vi "Dashboard Main.vi"() -> ()   [LabVIEW 2015]
uses:
  <vilib>/event_ctls.llb/eventvkey.ctl
  <vilib>/Rock Robotics/WPI/Dashboard/WPI_DashboardLogging Global.vi
  <vilib>/Rock Robotics/Network Tables/SD Read Number.vi
  <vilib>/Utility/config.llb/Write Key (String).vi
  <vilib>/Utility/config.llb/Write Key (I32).vi
  <vilib>/Utility/config.llb/NI_LVConfig.lvlib
panel:
  in  "TCP":refnum<k5>
  in  "Rec Mode":enum32{"Stop", "Record", "Playback"}(radio)
  in  "Vision":u16(ring) items=["Camera Off", "USB Camera SW", "USB Camera HW", "IP Camera"]
  out "Camera IP":string
  out "Image Message":string="Timeout in Camera Communications"
  in  "Dashboard Tab":T1(tab)
  out "TargetLocked":bool caption="Locked"
  out "AutoTarget":bool caption="Target\nTarget"
  out "ShooterLowPower":bool caption="Shoot Low"
  out "LSOverride":bool caption="LS OVR"
  out "PickupMotor":bool caption="Pickup"
  out "ShooterMotor":bool caption="Shooter"
  out "PTO":bool
  out "High":bool caption="High Gear"
  out "Low":bool caption="Low Gear"
  in  "CompressorEnabled":bool caption="Compressor"
  out "Compressor":bool
  in  "AutoProgramSelect":u16(ring) items=["0 - No Auto Program", "1 - Drive to Defense and Stop", "2 - Cross Rough Ground", "3 - Cross Rock Wall", "4 - Shoot from Spybot Start", "5 - Test Drive with Gyro"]
  out "Low Battery":bool
  out "FMS":bool
  out "Teleop Mode":bool
  out "Auto Mode":bool
  out "Disabled":bool
  in  "Program":string
  in  "Camera Settings":T2={"Frame Rate"=30, "Compression"=30, "Size"=1} {"Frame Rate" scale=1.0..30.0; "Size" items=["640x480", "320x240", "160x120"]}
  out "Mode":T3(ring)=enum."Auto Disabled"
  in  "DB Camera Config":bool
  out "fps":dbl format="%#.1g"
  out "Mbps":dbl format="%#.1g"
  out "Mbps 2":bool
  in  "PIDEnabled":bool caption="PID Enabled"
  in  "LCD_Line_10":string caption="DB/String 0"
  in  "LCD_Line_9":string caption="DB/String 0"
  in  "LCD_Line_8":string caption="DB/String 0"
  in  "LCD_Line_7":string caption="DB/String 0"
  in  "LCD_Line_6":string caption="DB/String 0"
  in  "LCD_Line_5":string caption="DB/String 0"
  in  "LCD_Line_4":string caption="DB/String 0"
  in  "LCD_Line_3":string caption="DB/String 0"
  in  "LCD_Line_2":string caption="DB/String 0"
  in  "LCD_Line_1":string caption="DB/String 0"
  in  "PValue":dbl caption="P"
  in  "IValue":dbl caption="I"
  in  "DValue":dbl caption="D"
  in  "LowSetting":dbl caption="Low"
  in  "HighSetting":dbl caption="High"
  in  "DB/String 9":string
  in  "DB/String 8":string
  in  "DB/String 7":string
  in  "DB/String 6":string
  in  "DB/String 5":string
  in  "DB/String 4":string
  in  "DB/String 3":string
  in  "DB/String 2":string
  in  "DB/String 1":string
  in  "DB/String 0":string
  in  "DB/Slider 0":dbl(slide) scale=0.0..5.0
  in  "DB/Slider 1":dbl(slide) scale=0.0..5.0
  in  "DB/Slider 2":dbl(slide) scale=0.0..5.0
  in  "DB/Slider 3":dbl(slide) scale=0.0..5.0
  out "DB/LED 3":bool
  out "DB/LED 2":bool
  out "DB/LED 1":bool
  out "DB/LED 0":bool
  in  "DB/Button 3":bool
  in  "DB/Button 2":bool
  in  "DB/Button 1":bool
  in  "DB/Button 0":bool caption="New Name"
  in  "Test Slider":dbl(slide) scale=0.0..100.0 scale format="%#_3g"
  in  "On/Off":bool caption="Solenoid"
  in  "Test Name":u16(ring) items=["Select the test to run...", "Example Test", "-------------------------------", "List of tests is built in robot code.", "Replace with your own automated tests."]
  in  "Test Tree":string(tree)
  in  "Motor":cluster{"Value":dbl, "Enable":bool} {"Value" scale=-1.0..1.0 scale format="%#_3g"}
  out "Progress":T4 {"Test Progress" scale=0.0..100.0}
  in  "Rev/Fwd":cluster{"Forward":bool, "Reverse":bool}
  in  "Test Ring":u16(ring) items=["Monochrome", "Color"]
  in  "Listbox":i32(listbox)
  out "Tree":string(tree)
  out "Camera Image":T5(plugin-control)
  out "Boolean":bool
  # "Program:"
  # "Dashboard: 2016-06"
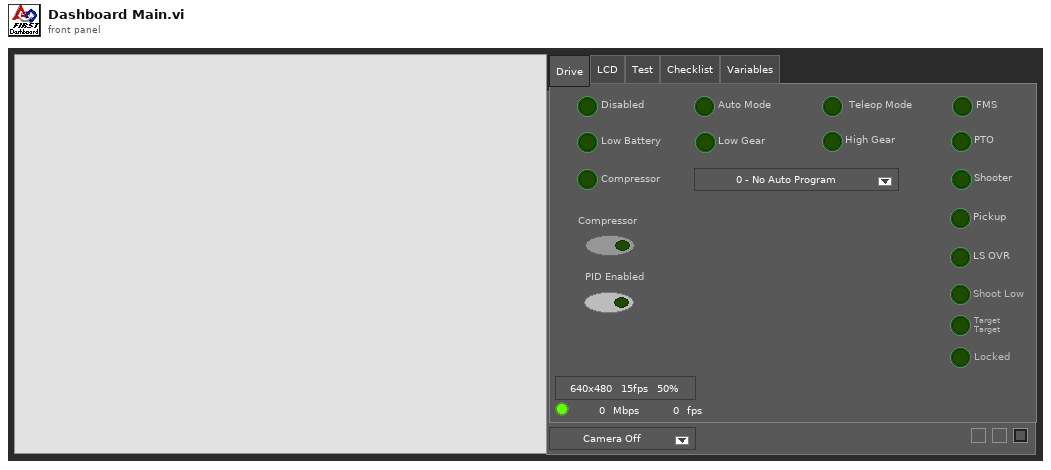
[diagram p1: front panel]
types:
  T1 = enum32{"Drive", "LCD", "Basic", "Test", "Checklist", "Variables"}
  T2 = cluster{"Frame Rate":i32, "Compression":i32, "Size":u16}
  T3 = enum8{"Tele-Op Disabled", "Tele-Op Enabled", "Auto Disabled", "Auto Enabled", "Test Disabled", "Test Enabled", "Disconnected", "No Code", "E-Stop"}
  T4 = cluster{"Test Progress":u8, "Test Progress Text":string}
  T5 = typedef "IMAQ Image.ctl" = refnum<image>
  T6 = enum32{"Drive", "Basic", "Custom", "Test", "Checklist", "Variables"}
  T7 = typedef "Image Type" = u32
  T8 = cluster{"Camera Image":refnum<vi>, "Dashboard Tab":refnum<vi>, "Boolean":refnum<vi>, "Vision":refnum<vi>, "Rec Mode":refnum<vi>, "Test Slider":refnum<vi>, "On/Off ":refnum<vi>, "Test Ring":refnum<vi>, "Rev/Fwd":refnum<vi>, "Test Name":refnum<vi>, "Motor":refnum<vi>, "Progress":refnum<vi>, "CheckList":refnum<vi>, "Tree":refnum<vi>, "Test Tree":refnum<vi>}
  T9 = cluster{"Error Strings":string, "Disable Counts":cluster{u16, u16}, "Rail Faults":cluster{u16, u16, u16}, "Robot IP":string, "DB Mode":u8, "Event Info":cluster{"Name":string, "Type":u8, "Number":u16, "Replay":u8}, "Camera Addr":string}
  T10 = cluster{"Storage":cluster{"Disk Free":u64, "RAM Block":u32, "RAM free":u32}, "CPU Utilization":cluster{"CPU % ISR":sgl, "CPU % Time Crit":sgl, "CPU % Timed Str":sgl, "CPU % High":sgl, "CPU % Above":sgl, "CPU % Normal":sgl, "CPU % Low":sgl}, "CAN":cluster{"% Bus Utilization":sgl, "Bus Off Cnt":u32, "TX_FIFO Full Cnt":u32, "Receive Error Cnt":u8, "Transmit Error Cnt":u8}, "HID":cluster{"HID Outputs":u32, "Rumble Low":u16, "Rumble High":u16}[]}
  T11 = cluster{"Status bits":cluster{"Test Mode":bool, "Autonomous":bool, "Enabled":bool, "Code Start":bool, "Brownout":bool, "Reserved 2":bool, "Reserved 3":bool, "E-Stop":bool}, "Code Trace":cluster{"Disabled":bool, "TeleOp":bool, "Auto":bool, "Test":bool}, "Controller Type":enum16{"unknown", "cRIO", "roboRio"}, "Code?":enum16{"unknown", "noCode", "code"}, "Battery V":dbl}
  T12 = cluster{"Control Bits":cluster{"TestMode":bool, "Autonomous":bool, "Enabled":bool, "FMS Present":bool, bool, bool, bool, "E-Stop":bool}, "Team Station ":u8, "Countdown":sgl, "Joystick Values":cluster{"Axes":dbl[], "Buttons":bool[], "POVs":i16[]}[]}
  T13 = cluster{"Axes":dbl[], "Buttons":bool[], "POVs":i16[]}[]
  T14 = cluster{"Axes":dbl[], "Buttons":bool[], "POVs":i16[]}
  T15 = typedef "NI_LVConfig.lvlib/Config Data RefNum.ctl" = refnum<k1>
  T16 = cluster{"Operation":enum16{"Update", "Clear"}, "Color Box":u32}[]
  T17 = typedef "eventvkey.ctl" = enum16{"ASCII", "Enter", "Return", "Shift", "Ctrl", "Alt", "Cmd", "Opt", "Caps", "NumLock", "Clear", "Break", "Up", "Down", "Left", "Right", "Insert", "Delete", "Home", "End", "PageUp", "PageDown", "Escape", "Help", "Pause", "ScrollLock", "F1", "F2", "F3", "F4", "F5", "F6", "F7", "F8", "F9", "F10", "F11", "F12", "F13", "F14", "F15", "F16", "F17", "F18", "F19", "F20", "F21", "F22", "F23", "F24", "Play", "VolumeUp", "VolumeDown", "Mute", "Two Byte Char"}
  T18 = cluster{"Image Size":bool, "Image Type":bool, "Pixel Value":bool, "ROI Information":bool, "Zoom Factor":bool}
  T19 = enum8{"Enabled", "Disabled", "Disabled and Grayed Out"}
  T20 = cluster{"Operation":enum16{"Update", "Clear"}, "Color Box":u32}
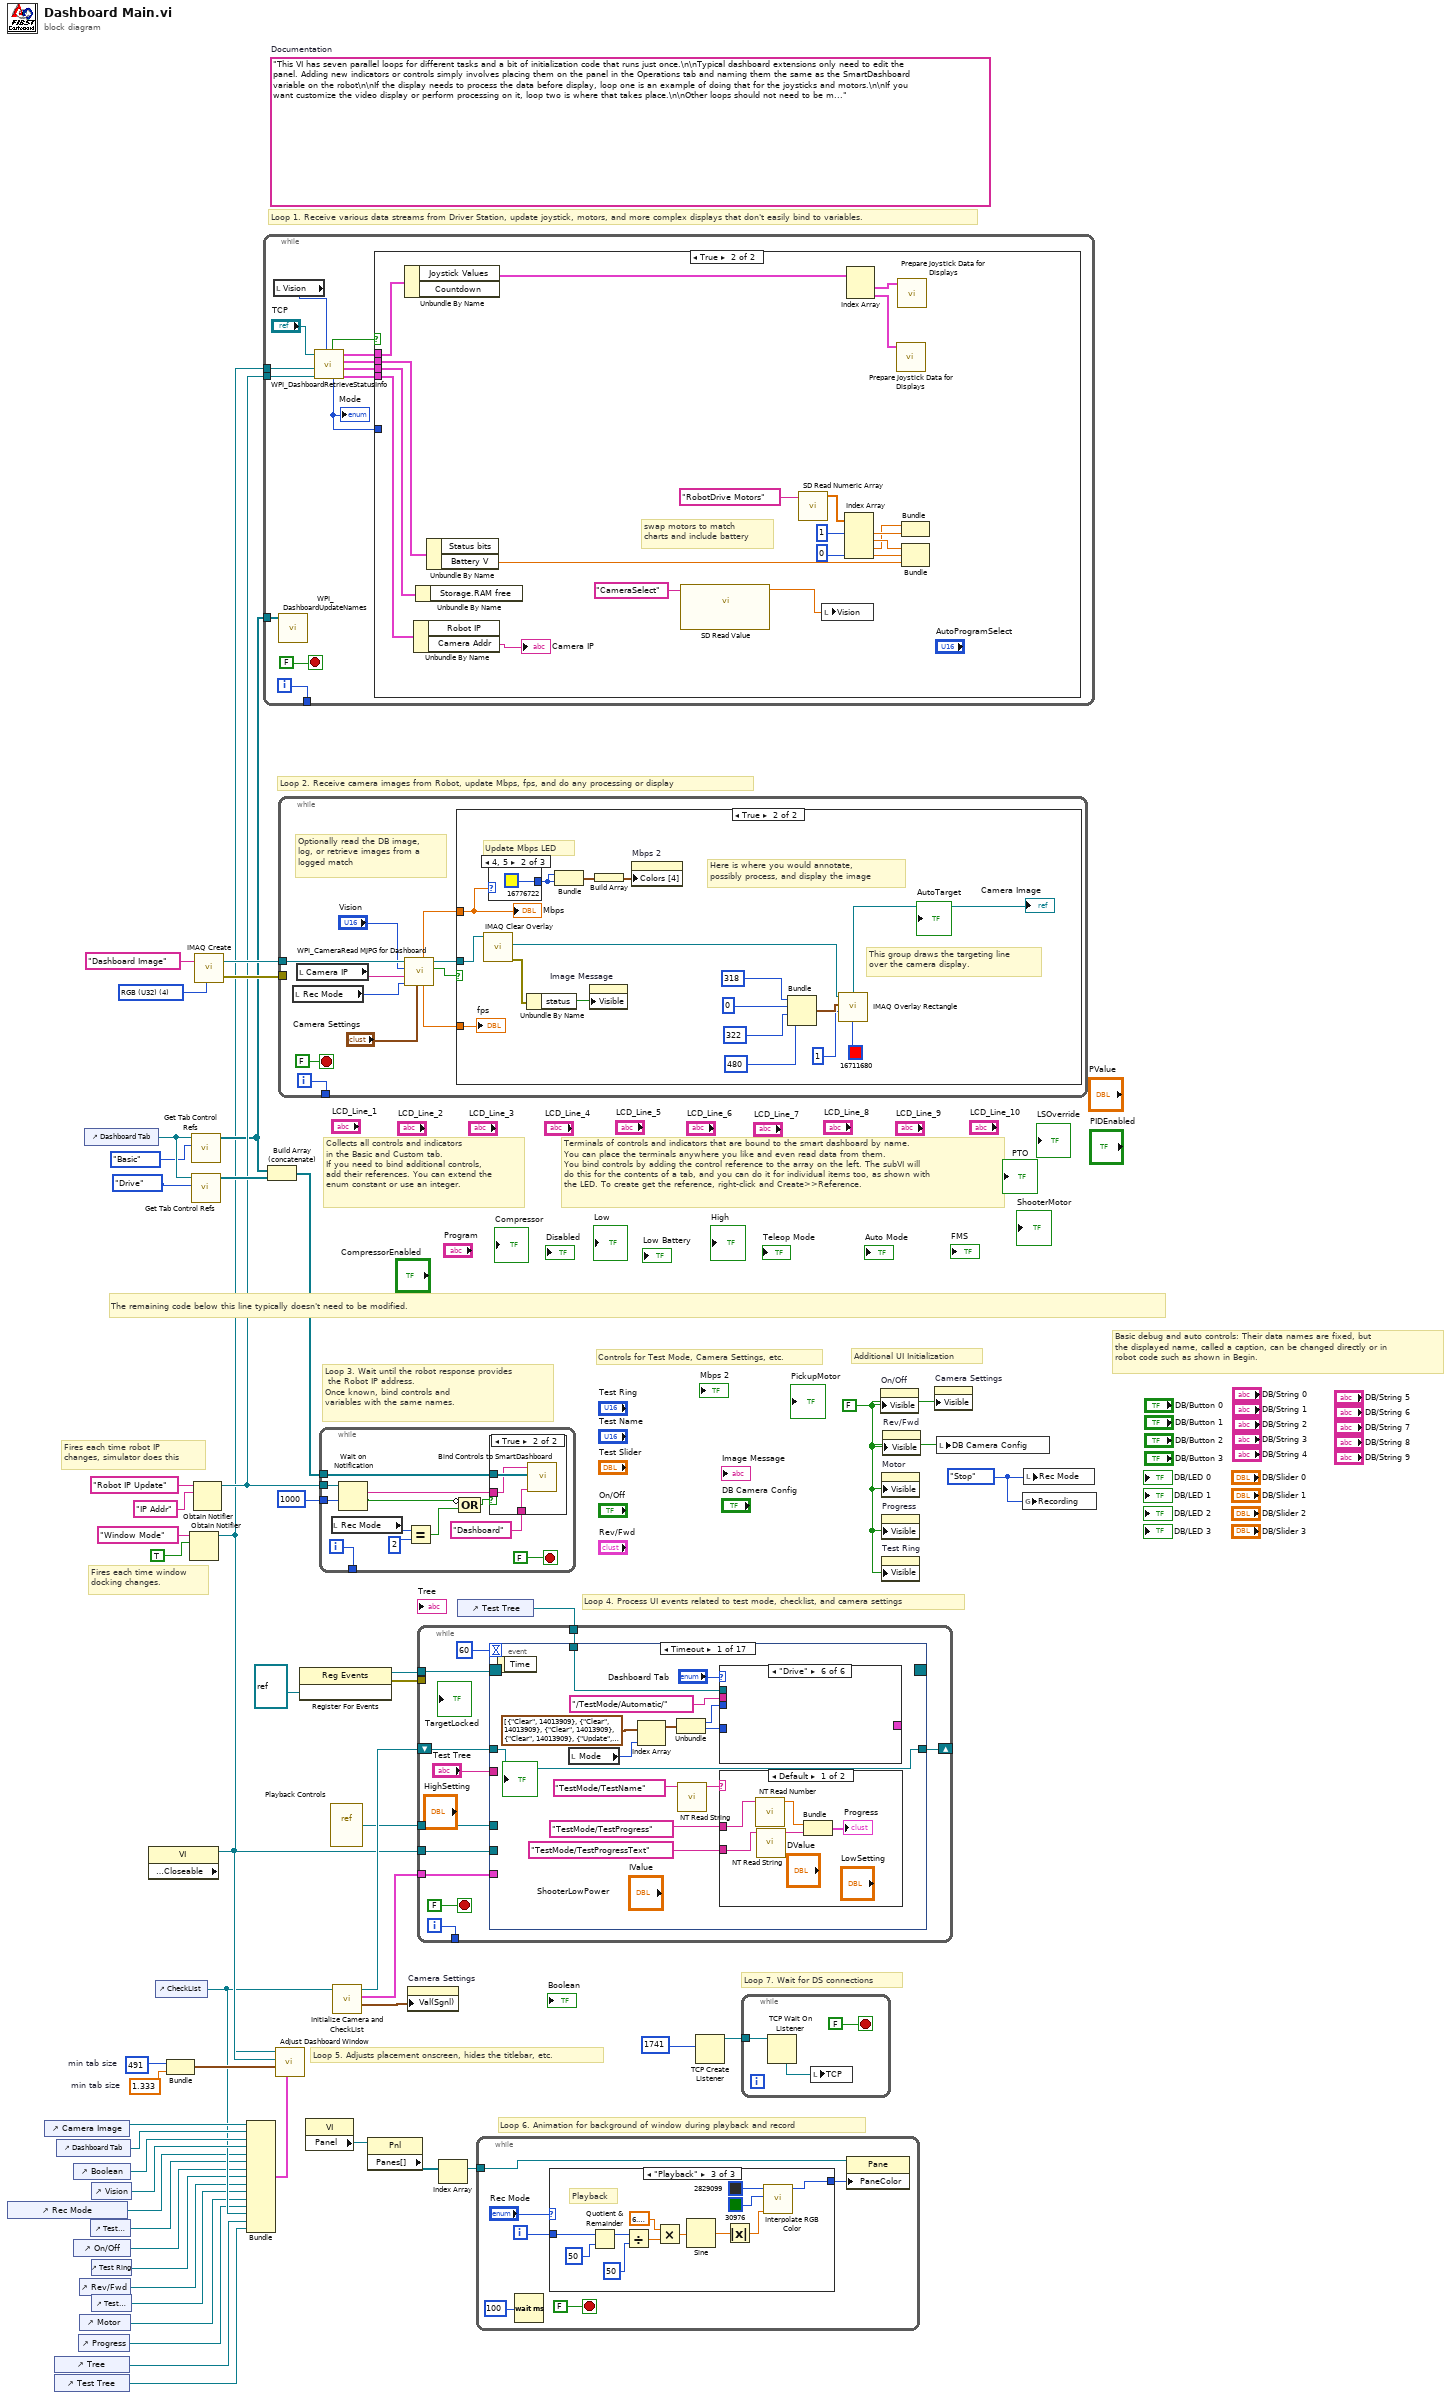
[diagram p0: block diagram]
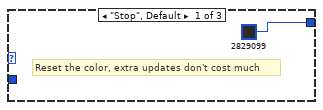
[diagram p3: hidden frame]
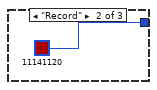
[diagram p4: hidden frame]
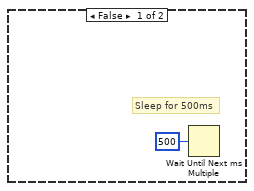
[diagram p6: hidden frame]
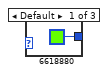
[diagram p7: hidden frame]
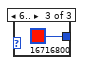
[diagram p8: hidden frame]
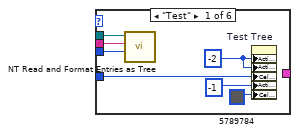
[diagram p9: hidden frame]
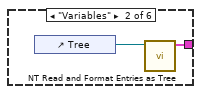
[diagram p10: hidden frame]
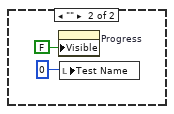
[diagram p14: hidden frame]
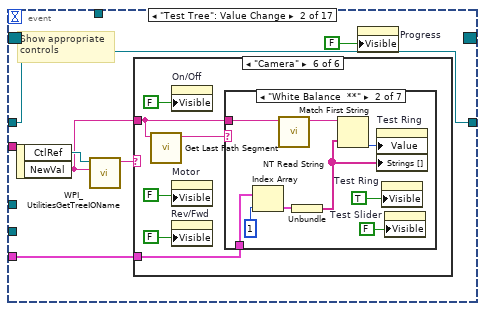
[diagram p15: hidden frame]
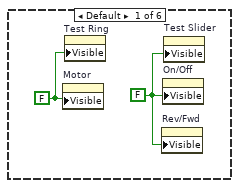
[diagram p16: hidden frame]
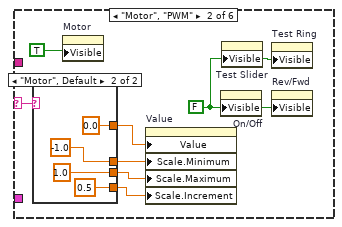
[diagram p17: hidden frame]
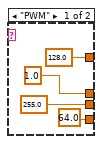
[diagram p18: hidden frame]
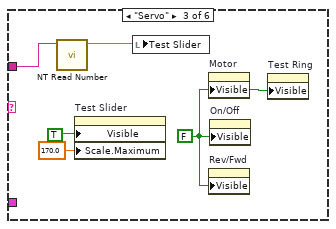
[diagram p19: hidden frame]
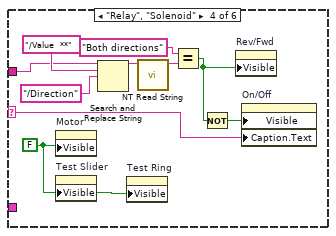
[diagram p20: hidden frame]
diagram:
  w24 = 491  # min tab size
  w23 = 1.333  # min tab size
  w32 = enum32{"Stop", "Record", "Playback"}."Stop" ("Rec Mode")
  w6 = FALSE ("Visible")
  (unwired) "This VI has seven parallel loops for different tasks and a bit of initialization code that runs just once.\n\nTypical dashboard extensions only need to edit the panel. Adding new indicators or controls simply involves placing them on the panel in the Operations tab and naming them the same as the SmartDashboard variable on the robot\n\nIf the display needs to process the data before display, loop one is an example of doing that for the joysticks and motors.\n\nIf you want customize the video display or perform processing on it, loop two is where that takes place.\n\nOther loops should not need to be modified. They are pretty standard, and document the task they perform."  # Documentation
  w52 = T7 4 items=["Grayscale (U8)", "Grayscale (I16)", "Grayscale (SGL)", "Complex (CSG)", "RGB (U32)", "HSL (U32)", "RGB (U64)"] ("Image Type")
  # "Loop 7. Wait for DS connections"
  # "Basic debug and auto controls: Their data names are fixed, but\nthe displayed name, called a caption, can be changed directly or in\nrobot code such as shown in Begin."
  # "Controls for Test Mode, Camera Settings, etc."
  # "Additional UI Initialization"
  # "Loop 6. Animation for background of window during playback and record"
  # "Fires each time robot IP\nchanges, simulator does this"
  # "Fires each time window\ndocking changes."
  # "Collects all controls and indicators\nin the Basic and Custom tab.\nIf you need to bind additional controls,\nadd their references. You can extend the\nenum constant or use an integer."
  # "The remaining code below this line typically doesn't need to be modified."
  # "Loop 4. Process UI events related to test mode, checklist, and camera settings"
  # "Terminals of controls and indicators that are bound to the smart dashboard by name.\nYou can place the terminals anywhere you like and even read data from them.\nYou bind controls by adding the control reference to the array on the left. The subVI will\ndo this for the contents of a tab, and you can do it for individual items too, as shown with\nthe LED. To create get the reference, right-click and Create>>Reference."
  # "Loop 3. Wait until the robot response provides\n the Robot IP address.\nOnce known, bind controls and\nvariables with the same names."
  # "Loop 5. Adjusts placement onscreen, hides the titlebar, etc."
  # "Loop 1. Receive various data streams from Driver Station, update joystick, motors, and more complex displays that don't easily bind to variables."
  # "Loop 2. Receive camera images from Robot, update Mbps, fps, and do any processing or display"
  n1 = control-ref of="Rec Mode"() -> (w12:refnum<vi>)
  n2 = control-ref of="Camera Image"() -> (w27:refnum<vi>)
  n3 = control-ref of="Tree"() -> (w16:refnum<vi>)
  n4 = control-ref of="Test Tree"() -> (w15:refnum<vi>)
  n5 = control-ref of="Dashboard Tab"() -> (w26:refnum<vi>)
  n6 = control-ref of="Boolean"() -> (w21:refnum<vi>)
  n7 = control-ref of="On/Off"() -> (w10:refnum<vi>)
  n8 = control-ref of="Progress"() -> (w7:refnum<vi>)
  n9 = control-ref of="Rev/Fwd"() -> (w8:refnum<vi>)
  n10 = control-ref of="Motor"() -> (w13:refnum<vi>)
  n11 = control-ref of="Dashboard Tab"() -> (w30:refnum<vi>)
  n12 = control-ref of="Test Slider"() -> (w11:refnum<vi>)
  n13 = control-ref of="Vision"() -> (w25:refnum<vi>)
  n14 = control-ref of="Test Ring"() -> (w9:refnum<vi>)
  n15 = control-ref of="Test Name"() -> (w14:refnum<vi>)
  n16 = property class="VI" props=["Front Panel.Closeable"]() -> (reference out=w31:refnum<vi>)  [unwired: 2 in, 2 out]
  n17 = control-ref of="CheckList"() -> (w17:refnum<vi>)
  n18 = Bundle("min tab size"=w24, "min tab size"=w23) -> (w22:cluster{"min tab size":i32, "min tab size":dbl})  [unwired: 1 in]
  n19 = Obtain Notifier(name (unnamed)="Window Mode", notification data type=TRUE) -> (notifier out=w3:refnum<notifier>)  [unwired: 2 in, 2 out]
  n20 = call <vilib>:"Get Tab Control Refs.vi"("Page Index"=T6."Basic" ("Dashboard Tab"), "TabControl in"=w30) -> ("ControlsOnPage"=w4:refnum<vi>[])  [unwired: 9 in]
  n21 = call <vilib>:"Get Tab Control Refs.vi"("Page Index"=T6."Drive" ("Dashboard Tab"), "TabControl in"=w30) -> ("ControlsOnPage"=w29:refnum<vi>[])  [unwired: 9 in]
  n22 = Obtain Notifier(name (unnamed)="Robot IP Update", notification data type="IP Addr" ("name (unnamed)")) -> (notifier out=w5:refnum<notifier>)  [unwired: 2 in, 2 out]
  n23 = call "IMAQ Create"("Image Name"="Dashboard Image", "Image Type"=w52) -> ("New Image"=w50:T5, "error out"=w49:errorcluster)  [unwired: 2 in, 1 out]
  n24 = Bundle("Camera Image"=w27, "Dashboard Tab"=w26, "Boolean"=w21, "Vision"=w25, "Rec Mode"=w12, "Test Slider"=w11, "On/Off"=w10, "Test Ring"=w9, "Rev/Fwd"=w8, "Test Name"=w14, "Motor"=w13, "Progress"=w7, "CheckList"=w17, "Tree"=w16, "Test Tree"=w15) -> (w18:T8)  [unwired: 1 in]
  n25 = while {
    tunnel: [w64] -> _
    tunnel: w5 -> [w58]
    tunnel: w4 -> [w57]
    tunnel: w3 -> [w53]
    i -> [w64]
    stop <- FALSE stop-if-true
    n26 = local read "Vision"() -> (w55:u16)
    n27 = call <vilib>:"WPI_DashboardUpdateNames.vi"("Controls on Tab"=w57) -> ()  [unwired: 11 in]
    n28 = call <vilib>:"WPI_DashboardRetrieveStatusInfo.vi"("Vision"=w55, "Binding Refnum"=w58, "Window Mode Notifier"=w53, "TCP Cnx"="TCP") -> ("Power and Errors"=w59:T9, "Robot Metrics"=w62:T10, "Status Info"=w63:T11, "Control Info"=w60:T12, "Robot Mode"=w56:T3, "Process?"=w61:bool)  [unwired: 2 in]
    "Mode" <- w56
    n29 = case shown="True" w61 {
      tunnel: w63 -> [_ w84]
      tunnel: w62 -> [_ w83]
      tunnel: w60 -> [_ w82]
      tunnel: w59 -> [_ w81]
      tunnel: w56 -> [_ _]
      frame False {
      }
      frame True {
        # "swap motors to match\ncharts and include battery"
        n30 = Unbundle By Name(w82) -> ("Joystick Values"=w71:T13)  [unwired: 1 out]
        n31 = Unbundle By Name(w81) -> ("Camera Addr"=→"Camera IP":string)  [unwired: 1 out]
        n32 = Unbundle By Name(w83) -> ()  [unwired: 1 out]
        n33 = Unbundle By Name(w84) -> ("Battery V"=w72:dbl)  [unwired: 1 out]
        n34 = call-poly <vilib>:"SD Read Value.vi"("Name"="CameraSelect") -> ("Numeric"=w67:dbl)  [unwired: 8 in, 2 out]
        n35 = call <vilib>:"SD Read Numeric Array.vi"("Name"="RobotDrive Motors") -> ("Numeric Array"=w74:dbl[])  [unwired: 8 in, 2 out]
        n36 = local write "Vision"(w67) -> ()
        n37 = Index Array(array=w74, index #1=1, index #4=0) -> (element #1=w76:dbl, element #2=w77:dbl, element #3=w75:dbl, element #4=w80:dbl)  [unwired: 2 in]
        n38 = Index Array(array=w71) -> (element #1=w70:T14, element #2=w68:T14)  [unwired: 2 in]
        n39 = call "Prepare Joystick Data for Displays.vi"("Joystick Values"=w68) -> ()  [unwired: 8 in, 3 out]
        n40 = call "Prepare Joystick Data for Displays.vi"("Joystick Values"=w70) -> ()  [unwired: 8 in, 3 out]
        n41 = Bundle("Numeric"=w75, "Numeric"=w76) -> ()  [unwired: 1 in, 1 out]
        n42 = Bundle("Numeric"=w77, "Numeric"=w80, "Battery V"=w72) -> ()  [unwired: 1 in, 1 out]
      }
    }
  }
  n43 = Build Array (concatenate)(w4, w29) -> (w28:refnum<vi>[])
  n44 = call "Adjust Dashboard Window.vi"("Sizing Refnums"=w18, "Size Constraints"=w22, "VI"=w31, "Notifier in"=w3) -> ()  [unwired: 8 in]
  n45 = while {
    tunnel: w50 -> [w93]
    tunnel: w49 -> [_]
    tunnel: [w94] -> _
    i -> [w94]
    stop <- FALSE stop-if-true
    # "Optionally read the DB image,\nlog, or retrieve images from a\nlogged match"
    n46 = local read "Rec Mode"() -> (w87:enum32{"Stop", "Record", "Playback"})
    n47 = local read "Camera IP"() -> (w85:string)
    n48 = call <vilib>:"WPI_CameraRead MJPG for Dashboard.vi"("Camera Settings"="Camera Settings", "Rec Mode"=w87, "Camera IP"=w85, "Camera Mode"="Vision", "Refnum in"=w93) -> ("Active"=w91:bool, "Refnum out"=w92:T5, "FPS"=w90:dbl, "Bandwidth (Mbps)"=w89:dbl)  [unwired: 3 in]
    n49 = case shown="True" w91 {
      tunnel: w92 -> [_ w108]
      tunnel: w89 -> [_ w107]
      tunnel: w90 -> [_ w106]
      frame False {
        # "Sleep for 500ms"
        n50 = Wait Until Next ms Multiple(millisecond multiple=u32 500) -> ()  [unwired: 1 out]
      }
      frame True {
        # "This group draws the targeting line\nover the camera display."
        # "Here is where you would annotate,\npossibly process, and display the image"
        # "Update Mbps LED"
        n51 = call "IMAQ Clear Overlay"("Image"=w108) -> ("error out"=w112:errorcluster, "Image Out"=w98:T5)  [unwired: 2 in, 7 out]
        n52 = case shown="4, 5" w107 {
          tunnel: [u32 6618880 ("Color Box") u32 16776722 ("Color Box") u32 16716800 ("Color Box")] -> w109
          frame Default {
          }
          frame 4, 5 {
          }
          frame 6.. {
          }
        }
        n53 = Unbundle By Name(w112) -> ("status"=w113:bool)
        n54 = Bundle("Color Box"=w109, "Color Box"=w109) -> (w111:cluster{"Color Box":u32, "Color Box":u32})  [unwired: 1 out]
        n55 = property on="Image Message" class="Str"("Visible"=w113) -> ()  [unwired: 2 in, 2 out]
        n56 = Build Array(w111) -> (w110:cluster{"Color Box":u32, "Color Box":u32}[])
        n57 = property on="Mbps 2" class="Bool (strict)"("Colors [4]"=w110) -> ()  [unwired: 2 in, 2 out]
        n58 = Bundle(318, 0, 322, 480) -> (w104:cluster{i32, i32, i32, i32})  [unwired: 1 out]
        n59 = call "IMAQ Overlay Rectangle"("Color"=u32 16711680, "Drawing Mode (Frame)"=1, "Rectangle"=w104, "Image"=w98) -> ("Image Out"=→"Camera Image":T5)  [unwired: 6 in, 1 out]
        "Mbps" <- w107
        "fps" <- w106
      }
    }
  }
  n60 = register-events(refnum<vi> refnum) -> (reference out=w36:refnum<event-registration>, error out=w35:errorcluster)  [unwired: 2 in]
  n61 = property class="VI"() -> ("Panel"=w39:refnum<vi>)  [unwired: 2 in, 2 out]
  n62 = while {
    tunnel: w28 -> [w128]
    tunnel: w5 -> [w126]
    tunnel: [w124] -> _
    tunnel: u32 1000 ("milliseconds to wait") -> [w123]
    i -> [w124]
    stop <- FALSE stop-if-true
    n63 = local read "Rec Mode"() -> (w119:enum32{"Stop", "Record", "Playback"})
    n64 = Wait on Notification(notifier=w126, timeout in ms (-1)=w123) -> (notification=w125:string, timed out?=w121:bool)  [unwired: 2 in, 2 out]
    n65 = Equal?(x=w119, y=u16 2 ("Rec Mode")) -> (x = y?=w120:bool)
    n66 = Compound Arithmetic op=OR(invert w121, w120) -> (w122:bool)
    n67 = case shown="True" w122 {
      tunnel: w128 -> [_ w131]
      tunnel: w125 -> [_ w130]
      tunnel: "Dashboard" -> [_ w129]
      frame False {
      }
      frame True {
        n68 = call <vilib>:"Bind Controls to SmartDashboard.vi"("Client Name"=w129, "Bound Control Refs"=w131, "Server IP Address"=w130) -> ()  [unwired: 9 in]
      }
    }
  }
  n69 = vi-ref "Playback Controls.vi"() -> (w37:refnum<vi>)
  n70 = call "Initialize Camera and CheckList.vi"("ListBox in"=w17) -> ("Cluster"=w43:cluster{"value":i32, "value":i32, "index":i32}, "Array"=w44:cluster{string[]}[], "File Refnum"=w42:T15)  [unwired: 8 in]
  n71 = property class="Pnl"(reference=w39) -> ("Panes[]"=w40:refnum<vi>[])  [unwired: 1 in, 2 out]
  n72 = property on="Camera Settings" class="Clust (strict)"("Val(Sgnl)"=w43) -> ()  [unwired: 2 in, 2 out]
  n73 = Index Array(array=w40) -> (element=w38:refnum<vi>)  [unwired: 1 in]
  n74 = control-ref of="Test Tree"() -> (w41:refnum<vi>)
  n75 = while {
    tunnel: w44 -> [w139]
    shift-right: [w138] -> _
    shift-left: w42 -> [w137]
    tunnel: [w136] -> _
    tunnel: w41 -> [w135]
    tunnel: w37 -> [w134]
    tunnel: w36 -> [w133]
    tunnel: w35 -> [_]
    tunnel: w31 -> [w132]
    i -> [w136]
    stop <- FALSE stop-if-true
    n76 = event shown="[0] Timeout" {
      selector: w133 -> [_ _ _ _ _ _ _ _ _ _ _ _ _ _ _ _ _]
      dyn-events: [_ _ _ _ _ _ _ _ _ _ _ _ _ w377 _ _ _] -> _
      timeout: u32 60 ("milliseconds to wait") -> [_ _ _ _ _ _ _ _ _ _ _ _ _ _ _ _ _]
      tunnel: w135 -> [w151 _ _ _ _ _ _ _ _ _ _ _ _ _ _ _ _]
      tunnel: "Test Tree" -> [_ _ _ _ _ _ _ _ w346 w354 w356 w360 w368 _ _ _ _]
      tunnel: w139 -> [_ w173 _ _ _ _ w310 w340 _ _ _ _ _ _ _ _ _]
      tunnel: [w147 w172 w271 w276 w284 w296 w309 w333 w345 w352 w355 w359 w367 w379 w393 w394 w404] -> w138
      tunnel: w137 -> [w147 w172 w271 w276 w284 w296 w308 w333 w345 w352 w355 w359 w367 w379 w393 w394 w404]
      tunnel: w134 -> [_ _ _ _ _ _ _ _ _ _ _ _ _ w380 _ w397 _]
      tunnel: w132 -> [_ _ _ _ _ _ _ _ _ _ _ _ _ w375 _ _ _]
      event Timeout {
        n77 = event-data() -> ()  [unwired: 1 in, 1 out]
        n78 = local read "Mode"() -> (w150:T3)
        n79 = Index Array(array=T16 [{"Operation"=enum."Clear", "Color Box"=14013909}, {"Operation"=enum."Clear", "Color Box"=14013909}, {"Operation"=enum."Clear", "Color Box"=14013909}, {"Operation"=enum."Clear", "Color Box"=14013909}, {"Operation"=enum."Update", "Color Box"=14013909}, {"Operation"=enum."Update", "Color Box"=16777215}, {"Operation"=enum."Clear", "Color Box"=14013909}, {"Operation"=enum."Clear", "Color Box"=14013909}, {"Operation"=enum."Clear", "Color Box"=14013909}], index=w150) -> (element=w145:T20)
        n80 = Unbundle(w145) -> ("Operation"=w144:enum16{"Update", "Clear"}, "Color Box"=w143:u32)
        n81 = call <vilib>:"NT Read String.vi"("Name"="TestMode/TestName") -> ("String"=w154:string)  [unwired: 9 in, 1 out]
        n82 = case shown="\"Drive\"" "Dashboard Tab" {
          tunnel: w151 -> [w162 _ _ _ _ _]
          tunnel: "/TestMode/Automatic/" ("Name Pattern") -> [w161 _ _ _ _ _]
          tunnel: w144 -> [w160 _ _ _ _ _]
          tunnel: [_ w164 _ _ _ _] -> _
          tunnel: w143 -> [w156 _ _ _ _ _]
          frame "Test" {
            w159 = -2 ("Active Item:Row Number")
            n83 = call <vilib>:"NT Read and Format Entries as Tree.vi"("Operation"=w160, "Name Pattern"=w161, "Tree Refnum"=w162) -> ()  [unwired: 7 in, 2 out]
            n84 = property on="Test Tree" class="Tree (strict)"("Active Item Row Number"=w159, "ActiveColNum"=w159, "CellBG"=w156, "Active Item Row Number"=-1 ("Active Item:Row Number"), "CellBG"=u32 5789784 ("Color Box")) -> ()  [unwired: 2 in, 2 out]
          }
          frame "Variables" {
            n85 = control-ref of="Tree"() -> (w163:refnum<vi>)
            n86 = call <vilib>:"NT Read and Format Entries as Tree.vi"("Tree Refnum"=w163) -> ("Formatted Strings"=w164:cluster{"Name":string, "Value":string}[])  [unwired: 9 in, 1 out]
          }
          frame "Checklist" {
          }
          frame "Basic" {
          }
          frame "LCD" {
          }
          frame "Drive" {
          }
        }
        n87 = case shown="Default" w154 {
          tunnel: "TestMode/TestProgress" ("Name") -> [w166 _]
          tunnel: "TestMode/TestProgressText" ("Name") -> [w165 _]
          frame Default {
            n88 = call <vilib>:"NT Read Number.vi"("Name"=w166) -> ("Numeric"=w167:dbl)  [unwired: 9 in, 1 out]
            n89 = call <vilib>:"NT Read String.vi"("Name"=w165) -> ("String"=w168:string)  [unwired: 9 in, 1 out]
            n90 = Bundle("Numeric"=w167, "String"=w168) -> (→"Progress":cluster{"Numeric":dbl, "String":string})  [unwired: 1 in]
          }
          frame "" {
            n91 = property on="Progress" class="Clust (strict)"("Visible"=FALSE) -> ()  [unwired: 2 in, 2 out]
            n92 = local write "Test Name"(u16 0) -> ()
          }
        }
      }
      event "Test Tree": Value Change {
        # "Show appropriate\ncontrols"
        n93 = event-data() -> ("CtlRef"=w176:refnum<vi>, "NewVal"=w174:string)  [unwired: 1 in]
        n94 = call <vilib>:"WPI_UtilitiesGetTreeIOName.vi"("NewVal"=w174, "TreeControl in"=w176) -> ("I/O Name"=w177:string)  [unwired: 9 in]
        n95 = case shown="\"Camera\"" w177 {
          selector: w177 -> [_ w184 _ w202 w211 _]
          tunnel: w174 -> [_ _ w199 w201 _ w218]
          tunnel: w173 -> [_ _ _ _ _ w217]
          frame Default {
            w179 = FALSE ("Visible")
            w178 = FALSE ("Visible")
            n96 = property on="Motor" class="Clust (strict)"("Visible"=w178) -> ()  [unwired: 2 in, 2 out]
            n97 = property on="Test Ring" class="Ring (strict)"("Visible"=w178) -> ()  [unwired: 2 in, 2 out]
            n98 = property on="Rev/Fwd" class="Clust (strict)"("Visible"=w179) -> ()  [unwired: 2 in, 2 out]
            n99 = property on="On/Off" class="Bool (strict)"("Visible"=w179) -> ()  [unwired: 2 in, 2 out]
            n100 = property on="Test Slider" class="Slide (strict)"("Visible"=w179) -> ()  [unwired: 2 in, 2 out]
          }
          frame "Motor", "PWM" {
            w185 = FALSE ("Visible")
            n101 = case shown="\"Motor\", Default" w184 {
              tunnel: [1.0 ("Value") -1.0 ("Value")] -> w183
              tunnel: [255.0 ("Value") 1.0 ("Value")] -> w182
              tunnel: [128.0 ("Value") 0.0 ("Value")] -> w181
              tunnel: [64.0 ("Value") 0.5 ("Value")] -> w180
              frame "PWM" {
              }
              frame "Motor", Default {
              }
            }
            n102 = property on="Motor" class="Clust (strict)"("Visible"=TRUE) -> ()  [unwired: 2 in, 2 out]
            n103 = property on="Value" class="Slide (strict)"("Value"=w181, "Scale.Minimum"=w183, "Scale.Maximum"=w182, "Scale.Increment"=w180) -> ()  [unwired: 2 in, 2 out]
            n104 = property on="On/Off" class="Bool (strict)"("Visible"=w185) -> ()  [unwired: 2 in, 2 out]
            n105 = property on="Test Slider" class="Slide (strict)"("Visible"=w185) -> ()  [unwired: 2 in, 2 out]
            n106 = property on="Test Ring" class="Ring (strict)"("Visible"=w185) -> ()  [unwired: 2 in, 2 out]
            n107 = property on="Rev/Fwd" class="Clust (strict)"("Visible"=w185) -> ()  [unwired: 2 in, 2 out]
          }
          frame "Servo" {
            w197 = FALSE ("Visible")
            n108 = call <vilib>:"NT Read Number.vi"("Name"=w199) -> ("Numeric"=w198:dbl)  [unwired: 9 in, 1 out]
            n109 = property on="Test Slider" class="Slide (strict)"("Visible"=TRUE, "Scale.Maximum"=170.0 ("Scale.Range:Maximum")) -> ()  [unwired: 2 in, 2 out]
            n110 = local write "Test Slider"(w198) -> ()
            n111 = property on="Motor" class="Clust (strict)"("Visible"=w197) -> ()  [unwired: 2 in, 2 out]
            n112 = property on="Rev/Fwd" class="Clust (strict)"("Visible"=w197) -> ()  [unwired: 2 in, 2 out]
            n113 = property on="On/Off" class="Bool (strict)"("Visible"=w197) -> ()  [unwired: 2 in, 2 out]
            n114 = property on="Test Ring" class="Ring (strict)"("Visible"=w197) -> ()  [unwired: 2 in, 2 out]
          }
          frame "Relay", "Solenoid" {
            w200 = FALSE ("Visible")
            n115 = property on="Motor" class="Clust (strict)"("Visible"=w200) -> ()  [unwired: 2 in, 2 out]
            n116 = property on="Test Slider" class="Slide (strict)"("Visible"=w200) -> ()  [unwired: 2 in, 2 out]
            n117 = Search and Replace String(input string=w201, search string="/Value  **", replace string="/Direction") -> (result string=w207:string)  [unwired: 5 in, 3 out]
            n118 = property on="Test Ring" class="Ring (strict)"("Visible"=w200) -> ()  [unwired: 2 in, 2 out]
            n119 = call <vilib>:"NT Read String.vi"("Name"=w207) -> ("String"=w205:string)  [unwired: 9 in, 1 out]
            n120 = Equal?(x="Both directions", y=w205) -> (x = y?=w203:bool)
            n121 = Not(x=w203) -> (.not. x?=w204:bool)
            n122 = property on="Rev/Fwd" class="Clust (strict)"("Visible"=w203) -> ()  [unwired: 2 in, 2 out]
            n123 = property on="On/Off" class="Bool (strict)"("Visible"=w204, "Caption.Text"=w202) -> ()  [unwired: 2 in, 2 out]
          }
          frame "Compressor", "Digital Out" {
            w210 = FALSE ("Visible")
            # "Get direction and finish"
            n124 = property on="Motor" class="Clust (strict)"("Visible"=w210) -> ()  [unwired: 2 in, 2 out]
            n125 = property on="Test Slider" class="Slide (strict)"("Visible"=w210) -> ()  [unwired: 2 in, 2 out]
            n126 = property on="Test Ring" class="Ring (strict)"("Visible"=w210) -> ()  [unwired: 2 in, 2 out]
            n127 = property on="On/Off" class="Bool (strict)"("Visible"=TRUE, "Caption.Text"=w211) -> ()  [unwired: 2 in, 2 out]
            n128 = property on="Rev/Fwd" class="Clust (strict)"("Visible"=FALSE) -> ()  [unwired: 2 in, 2 out]
          }
          frame "Camera" {
            n129 = call <vilib>:"Get Last Path Segment.vi"("String in"=w218) -> ("String out"=w219:string)  [unwired: 10 in]
            n130 = property on="On/Off" class="Bool (strict)"("Visible"=FALSE) -> ()  [unwired: 2 in, 2 out]
            n131 = property on="Motor" class="Clust (strict)"("Visible"=FALSE) -> ()  [unwired: 2 in, 2 out]
            n132 = property on="Rev/Fwd" class="Clust (strict)"("Visible"=FALSE) -> ()  [unwired: 2 in, 2 out]
            n133 = case shown="\"White Balance  **\"" w219 {
              tunnel: w218 -> [w225 w234 w243 w252 w261 _ w267]
              tunnel: w217 -> [w223 w231 w240 w249 w258 _ _]
              frame "Size  **" {
                n134 = Index Array(array=w223) -> (element=w222:cluster{string[]})  [unwired: 1 in]
                n135 = call <vilib>:"NT Read String.vi"("Name"=w225) -> ("String"=w224:string)  [unwired: 9 in, 1 out]
                n136 = Unbundle(w222) -> (w220:string[])
                n137 = Match First String(2:w220, 3:w224) -> (0:w221:i32)  [unwired: 1 out]
                n138 = property on="Test Ring" class="Ring (strict)"("Value"=w221, "Strings []"=w220) -> ()  [unwired: 2 in, 2 out]
                n139 = property on="Test Ring" class="Ring (strict)"("Visible"=TRUE) -> ()  [unwired: 2 in, 2 out]
                n140 = property on="Test Slider" class="Slide (strict)"("Visible"=FALSE) -> ()  [unwired: 2 in, 2 out]
              }
              frame "White Balance  **" {
                n141 = Index Array(array=w231, index=1) -> (element=w232:cluster{string[]})
                n142 = call <vilib>:"NT Read String.vi"("Name"=w234) -> ("String"=w233:string)  [unwired: 9 in, 1 out]
                n143 = Unbundle(w232) -> (w229:string[])
                n144 = Match First String(2:w229, 3:w233) -> (0:w228:i32)  [unwired: 1 out]
                n145 = property on="Test Ring" class="Ring (strict)"("Value"=w228, "Strings []"=w229) -> ()  [unwired: 2 in, 2 out]
                n146 = property on="Test Ring" class="Ring (strict)"("Visible"=TRUE) -> ()  [unwired: 2 in, 2 out]
                n147 = property on="Test Slider" class="Slide (strict)"("Visible"=FALSE) -> ()  [unwired: 2 in, 2 out]
              }
              frame "Exposure  **" {
                n148 = Index Array(array=w240, index=2) -> (element=w241:cluster{string[]})
                n149 = call <vilib>:"NT Read String.vi"("Name"=w243) -> ("String"=w242:string)  [unwired: 9 in, 1 out]
                n150 = Unbundle(w241) -> (w237:string[])
                n151 = Match First String(2:w237, 3:w242) -> (0:w238:i32)  [unwired: 1 out]
                n152 = property on="Test Ring" class="Ring (strict)"("Value"=w238, "Strings []"=w237) -> ()  [unwired: 2 in, 2 out]
                n153 = property on="Test Ring" class="Ring (strict)"("Visible"=TRUE) -> ()  [unwired: 2 in, 2 out]
                n154 = property on="Test Slider" class="Slide (strict)"("Visible"=FALSE) -> ()  [unwired: 2 in, 2 out]
              }
              frame "Exposure Priority  **" {
                n155 = Index Array(array=w249, index=3) -> (element=w250:cluster{string[]})
                n156 = call <vilib>:"NT Read String.vi"("Name"=w252) -> ("String"=w251:string)  [unwired: 9 in, 1 out]
                n157 = Unbundle(w250) -> (w246:string[])
                n158 = Match First String(2:w246, 3:w251) -> (0:w247:i32)  [unwired: 1 out]
                n159 = property on="Test Ring" class="Ring (strict)"("Value"=w247, "Strings []"=w246) -> ()  [unwired: 2 in, 2 out]
                n160 = property on="Test Ring" class="Ring (strict)"("Visible"=TRUE) -> ()  [unwired: 2 in, 2 out]
                n161 = property on="Test Slider" class="Slide (strict)"("Visible"=FALSE) -> ()  [unwired: 2 in, 2 out]
              }
              frame "Color Enable  **" {
                n162 = Index Array(array=w258, index=4) -> (element=w259:cluster{string[]})
                n163 = call <vilib>:"NT Read String.vi"("Name"=w261) -> ("String"=w260:string)  [unwired: 9 in, 1 out]
                n164 = Unbundle(w259) -> (w255:string[])
                n165 = Match First String(2:w255, 3:w260) -> (0:w256:i32)  [unwired: 1 out]
                n166 = property on="Test Ring" class="Ring (strict)"("Value"=w256, "Strings []"=w255) -> ()  [unwired: 2 in, 2 out]
                n167 = property on="Test Ring" class="Ring (strict)"("Visible"=TRUE) -> ()  [unwired: 2 in, 2 out]
                n168 = property on="Test Slider" class="Slide (strict)"("Visible"=FALSE) -> ()  [unwired: 2 in, 2 out]
              }
              frame Default {
                n169 = property on="Test Ring" class="Ring (strict)"("Visible"=FALSE) -> ()  [unwired: 2 in, 2 out]
                n170 = property on="Test Slider" class="Slide (strict)"("Visible"=FALSE) -> ()  [unwired: 2 in, 2 out]
              }
              frame "Brightness  **", "Color Level  **", "Compression  **", "FPS  **", "Sharpness  **" {
                n171 = call <vilib>:"NT Read Number.vi"("Name"=w267) -> ("Numeric"=w266:dbl)  [unwired: 9 in, 1 out]
                n172 = local write "Test Slider"(w266) -> ()
                n173 = property on="Test Slider" class="Slide (strict)"("Visible"=TRUE, "Scale.Maximum"=100.0 ("Scale.Range:Maximum")) -> ()  [unwired: 2 in, 2 out]
                n174 = property on="Test Ring" class="Ring (strict)"("Visible"=FALSE) -> ()  [unwired: 2 in, 2 out]
              }
            }
          }
        }
        n175 = property on="Progress" class="Clust (strict)"("Visible"=FALSE) -> ()  [unwired: 2 in, 2 out]
      }
      event "Test Name": Mouse Enter {
        # "Populate the ring with the list of tests"
        n176 = event-data() -> ()  [unwired: 1 in, 1 out]
        n177 = call <vilib>:"NT Read String Array.vi"("Name"="TestMode/TestList") -> ("String Array"=w275:string[])  [unwired: 9 in, 1 out]
        n178 = Build Array (concatenate)("Select the test to run...", w275) -> (w274:string[])
        n179 = property on="Test Name" class="Ring (strict)"("Strings []"=w274) -> ()  [unwired: 2 in, 2 out]
      }
      event "Test Name": Value Change {
        w277 = FALSE ("Visible")
        # "Tell the robot the test name to run"
        n180 = event-data() -> ("NewVal"=w281:u16)  [unwired: 1 in]
        n181 = property on="Test Name" class="Ring (strict)"() -> ("Strings []"=w282:string[])  [unwired: 2 in, 2 out]
        n182 = local write "Progress"(T4 {"Test Progress"=0, "Test Progress Text"=""} ("Progress")) -> ()
        n183 = Index Array(array=w282, index=w281) -> (element=w280:string)
        n184 = call <vilib>:"NT Write String.vi"("String"=w280, "Name"="TestMode/TestName") -> ()  [unwired: 9 in, 1 out]
        n185 = property on="Progress" class="Clust (strict)"("Visible"=TRUE) -> ()  [unwired: 2 in, 2 out]
        n186 = property on="Motor" class="Clust (strict)"("Visible"=w277) -> ()  [unwired: 2 in, 2 out]
        n187 = property on="Test Slider" class="Slide (strict)"("Visible"=w277) -> ()  [unwired: 2 in, 2 out]
        n188 = property on="On/Off" class="Bool (strict)"("Visible"=w277) -> ()  [unwired: 2 in, 2 out]
        n189 = property on="Rev/Fwd" class="Clust (strict)"("Visible"=w277) -> ()  [unwired: 2 in, 2 out]
        n190 = property on="Test Ring" class="Ring (strict)"("Visible"=w277) -> ()  [unwired: 2 in, 2 out]
      }
      event "Listbox": Double Click {
        # "Shift clears all"
        # "Update symbols on the listbox"
        n191 = event-data() -> ("PlatMods.Shift"=w285:bool, "Row"=w287:i32)  [unwired: 1 in]
        n192 = case shown="True" w285 {
          tunnel: w287 -> [w291 _]
          tunnel: 1 -> [w290 _]
          frame False {
            n193 = property on="Listbox" class="LstBox (strict)"() -> ("Item Symbols"=w289:i32[])  [unwired: 2 in, 2 out]
            n194 = Replace Array Subset(array=w289, new element=w290, index=w291) -> (w288:i32[])
            n195 = property on="Listbox" class="LstBox (strict)"("Item Symbols"=w288) -> ()  [unwired: 2 in, 2 out]
          }
          frame True {
            w292 = 0 ("Top Row")
            n196 = property on="Listbox" class="LstBox (strict)"() -> ("Number of Rows"=w294:u32)  [unwired: 2 in, 2 out]
            n197 = Initialize Array(0, w294) -> (w293:i32[])
            n198 = property on="Listbox" class="LstBox (strict)"("Top Row"=w292, "Value"=w292, "Item Symbols"=w293) -> ()  [unwired: 2 in, 2 out]
          }
        }
      }
      event "Listbox": Key Down {
        # "Update symbols on the listbox\nLeft and right keys check and uncheck"
        n199 = event-data() -> ("VKey"=w298:T17)  [unwired: 1 in]
        n200 = case shown="\"Left\", \"Right\"" w298 {
          selector: w298 -> [w303 _]
          tunnel: eventvkey."Left" ("VKey") -> [w301 _]
          frame "Left", "Right" {
            n201 = Equal?(x=w301, y=w303) -> (x = y?=w302:bool)
            n202 = Select(t=0, s=w302, f=1) -> (s? t:f=w304:i32)
            n203 = property on="Listbox" class="LstBox (strict)"() -> ("Item Symbols"=w307:i32[])  [unwired: 2 in, 2 out]
            n204 = Replace Array Subset(array=w307, new element=w304, index="Listbox") -> (w306:i32[])
            n205 = property on="Listbox" class="LstBox (strict)"("Item Symbols"=w306) -> ()  [unwired: 2 in, 2 out]
          }
          frame Default {
          }
        }
      }
      event "DB Camera Config": Value Change {
        # "Show or hide the cluster of controls, store in ini file"
        n206 = event-data() -> ("NewVal"=w311:bool)  [unwired: 1 in]
        n207 = case shown="False" w311 {
          tunnel: w310 -> [w320 _]
          tunnel: [w313 w331] -> w309
          tunnel: w308 -> [w312 w331]
          frame False {
            w327 = "Camera"
            w330 = FALSE ("Visible")
            n208 = local read "Camera Settings"() -> (w319:T2)
            n209 = Index Array(array=w320) -> (element=w323:cluster{string[]})  [unwired: 1 in]
            n210 = Unbundle(w319) -> ("Frame Rate"=w318:i32, "Compression"=w317:i32, "Size"=w321:u16)
            n211 = Unbundle(w323) -> (w322:string[])
            n212 = Index Array(array=w322, index=w321) -> (element=w316:string)
            n213 = call-poly <vilib>:"Write Key.vi"("section"=w327, "value"=w316, "key"="Size", "refnum"=w312) -> ("refnum out"=w329:T15)  [unwired: 2 in, 5 out]
            n214 = call-poly <vilib>:"Write Key.vi"("section"=w327, "value"=w318, "key"="FrameRate", "refnum"=w329) -> ("refnum out"=w328:T15)  [unwired: 1 in, 6 out]
            n215 = property on="Camera Settings" class="Clust (strict)"("Visible"=w330) -> ()  [unwired: 2 in, 2 out]
            n216 = local write "DB Camera Config"(w330) -> ()
            n217 = call-poly <vilib>:"Write Key.vi"("section"=w327, "value"=w317, "key"="Compression", "refnum"=w328) -> ("refnum out"=w314:T15)  [unwired: 1 in, 6 out]
            n218 = call <vilib>:"Close Config Data.vi"("refnum"=w314) -> ("file path"=w315:path)  [unwired: 2 in, 8 out]
            n219 = call <vilib>:"Open Config Data.vi"("configuration file path"=w315) -> ("refnum"=w313:T15)  [unwired: 8 in, 2 out]
          }
          frame True {
            n220 = property on="Camera Settings" class="Clust (strict)"("Visible"=TRUE) -> ()  [unwired: 2 in, 2 out]
          }
        }
      }
      event "Camera Settings": Value Change {
        # "Update summary string when any elements of DB camera change"
        n221 = event-data() -> ("NewVal"=w344:T2)  [unwired: 1 in]
        n222 = Index Array(array=w340) -> (element=w339:cluster{string[]})  [unwired: 1 in]
        n223 = Unbundle(w344) -> ("Frame Rate"=w335:i32, "Compression"=w334:i32, "Size"=w337:u16)
        n224 = Unbundle(w339) -> (w338:string[])
        n225 = Index Array(array=w338, index=w337) -> (element=w336:string)
        n226 = Format Into String(format string="%s   %dfps   %d%%", w336, w335, w334) -> (resulting string=w341:string)  [unwired: 2 in, 1 out]
        n227 = Build Array(w341) -> (w342:string[])
        n228 = property on="DB Camera Config" class="Bool (strict)"("Strings [4]"=w342) -> ()  [unwired: 2 in, 2 out]
      }
      event "Motor.Enable": Value Change {
        # "When the test mode otor enable helper is set, update that\ntree row item's value"
        n229 = event-data() -> ("NewVal"=w350:bool)  [unwired: 1 in]
        n230 = Unbundle("Motor") -> ("Value"=w349:dbl)  [unwired: 1 out]
        n231 = Select(t=w349, s=w350, f=0.0) -> (s? t:f=w347:dbl)
        n232 = call <vilib>:"NT Write Number.vi"("Numeric"=w347, "Name"=w346) -> ()  [unwired: 9 in, 1 out]
      }
      event "Test Slider": Value Change {
        # "When the test mode slider helper is set, update that\ntree row item's value"
        n233 = event-data() -> ("NewVal"=w353:dbl)  [unwired: 1 in]
        n234 = call <vilib>:"NT Write Number.vi"("Numeric"=w353, "Name"=w354) -> ()  [unwired: 9 in, 1 out]
      }
      event "On/Off": Value Change {
        # "When the test mode on/off helper value is set, update that\ntree row item's value"
        n235 = event-data() -> ("NewVal"=w358:bool)  [unwired: 1 in]
        n236 = Boolean To (0,1)(Boolean=w358) -> (0, 1=w357:i16)
        n237 = call <vilib>:"NT Write Number.vi"("Numeric"=w357, "Name"=w356) -> ()  [unwired: 9 in, 1 out]
      }
      event "Rev/Fwd": Value Change {
        # "When the test mode helper value for relays is set, update that\ntree row item's value"
        n238 = event-data() -> ("NewVal.Forward"=w366:bool, "NewVal.Reverse"=w365:bool)  [unwired: 1 in]
        n239 = Boolean To (0,1)(Boolean=w366) -> (0, 1=w362:i16)
        n240 = Boolean To (0,1)(Boolean=w365) -> (0, 1=w364:i16)
        n241 = Negate(x=w364) -> (-x=w363:i16)
        n242 = Add(x=w362, y=w363) -> (x+y=w361:i16)
        n243 = call <vilib>:"NT Write Number.vi"("Numeric"=w361, "Name"=w360) -> ()  [unwired: 9 in, 1 out]
      }
      event "Test Ring": Value Change {
        # "When a test mode helper value is selected from the ring,\nset the tree item's variable to the string value"
        n244 = event-data() -> ("NewVal"=w370:u16)  [unwired: 1 in]
        n245 = property on="Test Ring" class="Ring (strict)"() -> ("Strings []"=w371:string[])  [unwired: 2 in, 2 out]
        n246 = Index Array(array=w371, index=w370) -> (element=w369:string)
        n247 = call <vilib>:"NT Write String.vi"("String"=w369, "Name"=w368) -> ()  [unwired: 9 in, 1 out]
      }
      event "Rec Mode": Value Change {
        # "Update globals for recording mode and path to read log from.\nClear when logging and let NetworkTables set path for vision to\nuse."
        n248 = event-data() -> ("NewVal"=w381:enum32{"Stop", "Record", "Playback"})  [unwired: 1 in]
        n249 = global write "WPI_DashboardLogging Global.vi" "Logging Filename"(path "") -> ()
        n250 = case shown="\"Playback\"" w381 {
          tunnel: w380 -> [_ w383 w391]
          tunnel: [_ _ w390] -> w377
          tunnel: [_ _ w389] -> _
          tunnel: w375 -> [_ _ w387]
          tunnel: cluster{i32, i32} {-250, 170} -> [_ _ w386]
          tunnel: [_ _ T18 {"Image Size"=TRUE, "Image Type"=TRUE, "Pixel Value"=TRUE, "ROI Information"=TRUE, "Zoom Factor"=FALSE} ("Image Information Shown:All Elements")] -> w373
          tunnel: [_ _ TRUE ("Zoom Factor")] -> w372
          frame Default {
          }
          frame "Stop", "Record" {
            # "Place Window too"
            n251 = invoke class="VI" method="FP.Close"(reference=w383) -> (reference out=w382:refnum<vi>)  [unwired: 2 in, 2 out]
            n252 = invoke class="VI" method="Abort VI"(reference=w382) -> ()  [unwired: 2 in, 3 out]
          }
          frame "Playback" {
            n253 = call "Open Playback Panel.vi"("Offset"=w386, "DB VI Ref"=w387, "Playback in"=w391) -> ("Playback out"=w388:refnum<vi>)  [unwired: 8 in]
            n254 = register-events(w388) -> (reference out=w390:refnum<event-registration>, error out=w389:errorcluster)  [unwired: 2 in]
          }
        }
        n255 = global write "WPI_DashboardLogging Global.vi" "Recording"(w381) -> ()
        n256 = property on="Camera Image" class="ImageControl"("Image Information Shown"=w373, "Image Information Visible"=w372) -> ()  [unwired: 2 in, 2 out]
        n257 = call <vilib>:"WPI_DashboardNT Log FieldName Cache.vi"("Operation"=enum16{"Lookup/Add", "Index", "Clear"}."Clear") -> ()  [unwired: 8 in, 3 out]
      }
      event Panel Close {
        w392 = enum32{"Stop", "Record", "Playback"}."Stop" ("Rec Mode")
        # "Playback window has been closed, abort"
        n258 = event-data() -> ()  [unwired: 1 in, 4 out]
        n259 = local write "Rec Mode"(w392) -> ()
        n260 = global write "WPI_DashboardLogging Global.vi" "Recording"(w392) -> ()
      }
      event Panel Close {
        # "Abort playback window and ourself"
        n261 = event-data() -> ()  [unwired: 1 in, 4 out]
        n262 = invoke class="VI" method="FP.Close"(reference=w397) -> (reference out=w396:refnum<vi>)  [unwired: 2 in, 2 out]
        n263 = invoke class="VI" method="Abort VI"(reference=w396) -> (error out=w395:errorcluster)  [unwired: 2 in, 2 out]
        n264 = invoke class="VI" method="Abort VI"(error in=w395) -> ()  [unwired: 2 in, 3 out]
      }
      event "Vision": Value Change {
        # "Enable/Disable Compression slider.\nHW USB is hard-coded into the camera"
        n265 = event-data() -> ("NewVal"=w403:u16)  [unwired: 1 in]
        n266 = Equal?(x=w403, y=u32 2 ("milliseconds to wait")) -> (x = y?=w401:bool)
        n267 = Select(t=T19."Disabled and Grayed Out" ("Disabled"), s=w401, f=T19."Enabled" ("Disabled")) -> (s? t:f=w398:T19)
        n268 = property on="Compression" class="Slide (strict)"("DisabledEnum"=w398) -> ()  [unwired: 2 in, 2 out]
      }
    }
  }
  n269 = while {
    tunnel: w38 -> [w406]
    i -> [w409]
    stop <- FALSE stop-if-true
    n270 = Wait (ms)(milliseconds to wait=u32 100) -> ()  [unwired: 1 out]
    n271 = case shown="\"Playback\"" "Rec Mode" {
      tunnel: w409 -> [_ _ w424]
      tunnel: [u32 2829099 ("Base Color") u32 11141120 ("Target Color") w413] -> w405
      frame "Stop", Default {
        # "Reset the color, extra updates don't cost much"
      }
      frame "Record" {
      }
      frame "Playback" {
        # "Playback"
        n272 = Quotient & Remainder(x=w424, y=u32 50 ("milliseconds to wait")) -> (x-y*floor(x/y)=w420:u32)  [unwired: 1 out]
        n273 = Divide(x=w420, y=u32 50 ("milliseconds to wait")) -> (x/y=w417:dbl)
        n274 = Multiply(x=6.283185307179586, y=w417) -> (x*y=w422:dbl)
        n275 = Sine(x=w422) -> (sin(x)=w421:dbl)
        n276 = Absolute Value(x=w421) -> (abs(x)=w414:dbl)
        n277 = call "Interpolate RGB Color.vi"("Proportion"=w414, "Target Color"=u32 30976, "Base Color"=u32 2829099) -> ("Result Color"=w413:u32)  [unwired: 8 in]
      }
    }
    n278 = property class="Pane"(reference=w406, "PaneColor"=w405) -> ()  [unwired: 1 in, 2 out]
  }
  n279 = TCP Create Listener(10:u16 1741 ("timeout ms (25000)")) -> (3:w1:refnum<k5>)  [unwired: 4 in, 2 out]
  n280 = while {
    tunnel: w1 -> [w426]
    stop <- FALSE stop-if-true
    n281 = TCP Wait On Listener(11:w426) -> (4:w425:refnum<k5>)  [unwired: 3 in, 4 out]
    n282 = local write "TCP"(w425) -> ()
  }
  n283 = property on="On/Off" class="Bool (strict)"("Visible"=w6) -> ()  [unwired: 2 in, 2 out]
  n284 = property on="Motor" class="Clust (strict)"("Visible"=w6) -> ()  [unwired: 2 in, 2 out]
  n285 = property on="Progress" class="Clust (strict)"("Visible"=w6) -> ()  [unwired: 2 in, 2 out]
  n286 = property on="Test Ring" class="Ring (strict)"("Visible"=w6) -> ()  [unwired: 2 in, 2 out]
  n287 = property on="Rev/Fwd" class="Clust (strict)"("Visible"=w6) -> ()  [unwired: 2 in, 2 out]
  n288 = property on="Camera Settings" class="Clust (strict)"("Visible"=w6) -> ()  [unwired: 2 in, 2 out]
  n289 = local write "DB Camera Config"(w6) -> ()
  n290 = global write "WPI_DashboardLogging Global.vi" "Recording"(w32) -> ()
  n291 = local write "Rec Mode"(w32) -> ()
